vi "Configure Measurement (Time Interval Error).vi"(0 "VISA resource name":refnum<visa-resource-name>, 1 "Direction (0: Rising)":i32(ring) items=["Rising", "Falling", "Both"], 2 "Units (0: Second)":i32(ring) items=["Second", "Unit Interval"], 5 "Measurement Source (1: Channel 1)":i32(ring)=1 caption="Channel (1: Channel 1)" items=["Channel 1"=1, "Channel 2"=2, "Channel 3"=3, "Channel 4"=4, "Function 1"=5, "Function 2"=6, "Function 3"=7, "Function 4"=8, "Memory 1"=9, "Memory 2"=10, "Memory 3"=11, "Memory 4"=12, "Clock"=15, "MTrend"=16, "MSpectrum"=17, "Equalized"=18, "DIG 0"=20, "DIG 1"=21, "DIG 2"=22, "DIG 3"=23, "DIG 4"=24, "DIG 5"=25, "DIG 6"=26, "DIG 7"=27, "DIG 8"=28, "DIG 9"=29, "DIG 10"=30, "DIG 11"=31, "DIG 12"=32, "DIG 13"=33, "DIG 14"=34, "DIG 15"=35], 9 "Measurement Function (0: Time Interval Error (Data))":i32(ring) items=["Time Interval Error (Data)", "Time Interval Error (Clock)"], 11 "error in (no error)":errorcluster) -> (4 "VISA resource name out":refnum<visa-resource-name>, 15 "error out":errorcluster)   [LabVIEW 2013, in "Agilent 90000 Series.lvlib"]
doc: "Configures time interval error measurement.\n\n<B>Note:</B>\nCalling this VI disables all previously enabled measurements and clears existing measurement results from display."
uses:
  Agilent 90000 Series.lvlib
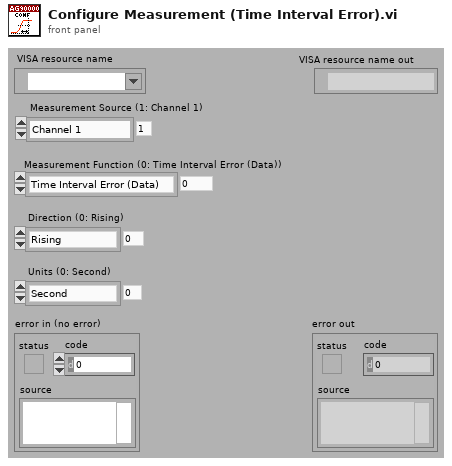
[diagram p1: front panel]
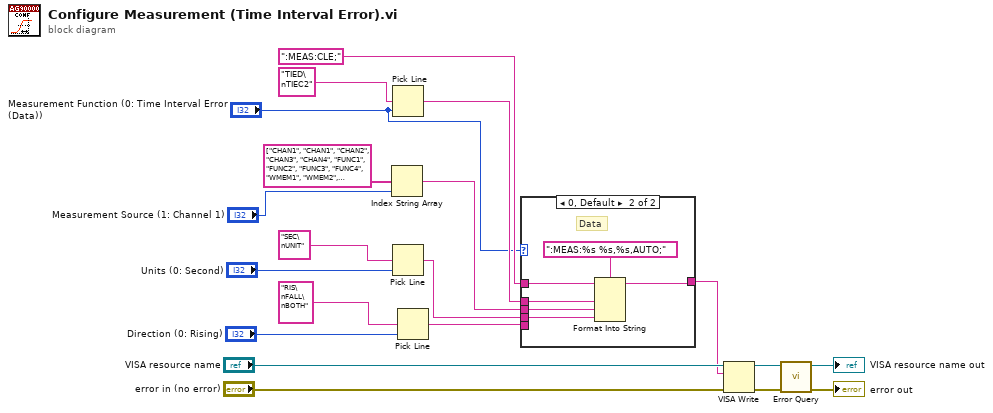
[diagram p0: block diagram]
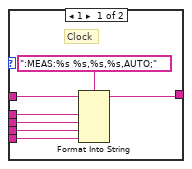
[diagram p2: hidden frame]
diagram:
  n1 = Index String Array(1:"Measurement Source (1: Channel 1)", 2:string[] ["CHAN1", "CHAN1", "CHAN2", "CHAN3", "CHAN4", "FUNC1", "FUNC2", "FUNC3", "FUNC4", "WMEM1", "WMEM2", "WMEM3", "WMEM4", "AUX", "LINE", "CLOC", "MTR", "MSP", "EQU", "NONE", "DIG0", "DIG1", "DIG2", "DIG3", "DIG4", "DIG5", "DIG6", "DIG7", "DIG8", "DIG9", "DIG10", "DIG11", "DIG12", "DIG13", "DIG14", "DIG15", "", "", "", "", "", "POD1", "POD2", "", "", "", "", "", "", "", "", "BUS1", "BUS2", "BUS3", "BUS4", "", "", "", "", "", "", "DIFF1", "DIFF2", "", "", "", "", "", "", "", "", "COMM3", "COMM4"]) -> (0:w11:string)  [unwired: 1 out]
  n2 = Pick Line(multi-line string="TIED\nTIEC2", line index="Measurement Function (0: Time Interval Error (Data))") -> (output string=w12:string)  [unwired: 1 out]
  n3 = Pick Line(multi-line string="SEC\nUNIT", line index="Units (0: Second)") -> (output string=w5:string)  [unwired: 1 out]
  n4 = Pick Line(multi-line string="RIS\nFALL\nBOTH", line index="Direction (0: Rising)") -> (output string=w4:string)  [unwired: 1 out]
  n5 = case shown="0, Default" "Measurement Function (0: Time Interval Error (Data))" {
    tunnel: ":MEAS:CLE;" ("initial string") -> [w27 w33]
    tunnel: w12 -> [w25 w31]
    tunnel: w11 -> [w24 w30]
    tunnel: [w23 w29] -> w3
    tunnel: w5 -> [w22 w28]
    tunnel: w4 -> [w21 _]
    frame 1 {
      # "Clock"
      n6 = Format Into String(format string=":MEAS:%s %s,%s,%s,AUTO;", initial string=w27, w25, w24, w22, w21) -> (resulting string=w23:string)  [unwired: 1 in, 1 out]
    }
    frame 0, Default {
      # "Data"
      n7 = Format Into String(format string=":MEAS:%s %s,%s,AUTO;", initial string=w33, w31, w30, w28) -> (resulting string=w29:string)  [unwired: 1 in, 1 out]
    }
  }
  n8 = VISA Write(VISA resource name="VISA resource name", write buffer=w3, error in (no error)="error in (no error)") -> (VISA resource name out=w16:refnum<visa-resource-name>, error out=w15:errorcluster)  [unwired: 1 out]
  n9 = call "Error Query.vi"("error in (no error)"=w15, "VISA resource name"=w16) -> ("error out"=→"error out":errorcluster, "VISA resource name out"=→"VISA resource name out":refnum<visa-resource-name>)  [unwired: 8 out]
